vi "SIAM_test_Standalone.vi"() -> ()   [LabVIEW 2011]
uses:
  SIAM_command.ctl
  Library/ScanControl/ScanControl_Action.ctl
  Library/ScanControl/ScanControl_Channel.ctl
  SIAM-send.ctl
  <vilib>/Utility/miscctls.llb/LVRangeTypeDef.ctl
panel:
  in  "Registerkarte":enum32{"Config", "Scan", "Work", "Debug"}(tab)
  out "Instrument check":bool
  in  "expected instrument name":string="Earn_Out"
  in  "TMSI-device-scales":T2(array[cluster])=[{"channel"=enum."GalvoX", "m/bit"=8e-07, "min m"=-0.01, "max m"=0.01, "max a [m/s]"=1.0}, {"channel"=enum."GalvoY", "m/bit"=8e-07, "min m"=-0.01, "max m"=0.01, "max a [m/s]"=1.0}, {"channel"=enum."Galvo3", "m/bit"=2e-09, "min m"=-0.01, "max m"=0.02, "max a [m/s]"=1.0}]
  out "Connected":bool
  in  "remote port or service name":u16=3
  in  "address":string="10.153.70.119"
  out "connect error":errorcluster
  in  "Cycletime [s]":dbl=1e-05
  in  "Update length":bool
  out "Elements":i32
  in  "Unroll-loops":bool
  in  "ClearScan":bool
  in  "channel":T1=enum."GalvoX"
  in  "ConvertScan":bool
  in  "Convert String":bool
  in  "Colibri-Scan-String":string="0,0,10,0.00119;0,0,3,-7.2266666667E-5;0,0,4,-8.8133333333E-5;0,0,11,0;0,0,12,0;0,0,7,3;0,4,9,127;0,2,3,0.05875;0,2,4,0;0,2,11,100000;0.00255,2,11,0;0.00256,1,12,1;0.00256,0,7,1;0.00256,2,3,-1.4928955695E-16;0.00256,2,4,0.0073046875;0.00264,0,7,3;0.00264,2,3,-0.05875;0.00264,2,4,0;0.00264,2,11,-100000;0.00519,2,11,0;0.0052,1,12,1;0.0052,0,7,1;0.0052,2,3,1.4928955695E-16;0.0052,2,4,0.0073046875;0.00528,0,7,3;0.00528,5,9,0;0.67056,2,3,0.05875;0.67056,2,4,0;0.67056,2,11,100000;0.67311,2,11,0;0.67312,1,12,1;0.67312,0,7,1;0.67312,2,3,-1.4928955695E-16;0.67312,2,4,0.0073046875;0.6732,0,7,3;0.6732,2,3,-0.05875;0.6732,2,4,0;0.6732,2,11,-100000;0.67575,2,11,0;0.67576,2,3,0;0.67576,2,4,0;0.67576,0,7,0;"
  in  "ScanSteuerung":T4(array[cluster])
  in  "Frequency [Hz]":dbl=500.0
  in  "duration [s]":dbl=1.0
  in  "Amplitude (count pk-pk)":dbl=6553.6 format="%#_5g"
  in  "Create":bool
  in  "Offset [count]":dbl=1.0
  in  "Run":bool
  in  "SendScript":bool
  in  "Load":bool
  in  "Save":bool
  in  "ClearScript":bool
  in  "Value":i32
  in  "Motor":T5(ring)
  in  "Position":i32(slide)
  in  "Clear":bool
  in  "Special":bool
  in  "return":string
  in  "special send options":T6
  in  "Script":T8(array[cluster])=[{"Delay 10µs"=0, "command"=100663297, "P0"=1024, "P1"=-2147483648, "P2"=0, "P3"=0, "P4"=0, "P5-ticket"=0}, {"Delay 10µs"=0, "command"=100663297, "P0"=16384, "P1"=2147483647, "P2"=0, "P3"=0, "P4"=0, "P5-ticket"=0}, {"Delay 10µs"=0, "command"=100663297, "P0"=512, "P1"=2147483647, "P2"=0, "P3"=0, "P4"=0, "P5-ticket"=0}, {"Delay 10µs"=0, "command"=100663297, "P0"=8192, "P1"=0, "P2"=0, "P3"=0, "P4"=0, "P5-ticket"=0}, {"Delay 10µs"=119, "command"=4060086273, "P0"=2, "P1"=99, "P2"=0, "P3"=0, "P4"=0, "P5-ticket"=0}, {"Delay 10µs"=0, "command"=218103809, "P0"=255, "P1"=7, "P2"=0, "P3"=0, "P4"=0, "P5-ticket"=0}, {"Delay 10µs"=281, "command"=100663297, "P0"=512, "P1"=0, "P2"=0, "P3"=0, "P4"=0, "P5-ticket"=0}, {"Delay 10µs"=0, "command"=100663297, "P0"=8192, "P1"=-2147483648, "P2"=0, "P3"=0, "P4"=0, "P5-ticket"=0}, {"Delay 10µs"=8, "command"=100663297, "P0"=512, "P1"=-2147483648, "P2"=0, "P3"=0, "P4"=0, "P5-ticket"=0}, {"Delay 10µs"=0, "command"=100663297, "P0"=8192, "P1"=0, "P2"=0, "P3"=0, "P4"=0, "P5-ticket"=0}, {"Delay 10µs"=111, "command"=218103809, "P0"=255, "P1"=5, "P2"=0, "P3"=0, "P4"=0, "P5-ticket"=0}, {"Delay 10µs"=8, "command"=218103809, "P0"=255, "P1"=7, "P2"=0, "P3"=0, "P4"=0, "P5-ticket"=0}, {"Delay 10µs"=281, "command"=100663297, "P0"=512, "P1"=0, "P2"=0, "P3"=0, "P4"=0, "P5-ticket"=0}, {"Delay 10µs"=0, "command"=100663297, "P0"=8192, "P1"=-2147483648, "P2"=0, "P3"=0, "P4"=0, "P5-ticket"=0}, {"Delay 10µs"=8, "command"=100663297, "P0"=512, "P1"=2147483647, "P2"=0, "P3"=0, "P4"=0, "P5-ticket"=0}, {"Delay 10µs"=0, "command"=100663297, "P0"=8192, "P1"=0, "P2"=0, "P3"=0, "P4"=0, "P5-ticket"=0}, {"Delay 10µs"=111, "command"=218103809, "P0"=255, "P1"=5, "P2"=0, "P3"=0, "P4"=0, "P5-ticket"=0}, {"Delay 10µs"=8, "command"=4043375201, "P0"=-12, "P1"=2, "P2"=1, "P3"=0, "P4"=0, "P5-ticket"=0}, {"Delay 10µs"=0, "command"=218103809, "P0"=255, "P1"=7, "P2"=0, "P3"=0, "P4"=0, "P5-ticket"=0}, {"Delay 10µs"=281, "command"=100663297, "P0"=512, "P1"=0, "P2"=0, "P3"=0, "P4"=0, "P5-ticket"=0}, {"Delay 10µs"=0, "command"=100663297, "P0"=8192, "P1"=-2147483648, "P2"=0, "P3"=0, "P4"=0, "P5-ticket"=0}, {"Delay 10µs"=8, "command"=100663297, "P0"=512, "P1"=-2147483648, "P2"=0, "P3"=0, "P4"=0, "P5-ticket"=0}, {"Delay 10µs"=0, "command"=100663297, "P0"=8192, "P1"=0, "P2"=0, "P3"=0, "P4"=0, "P5-ticket"=0}, {"Delay 10µs"=111, "command"=218103809, "P0"=255, "P1"=5, "P2"=0, "P3"=0, "P4"=0, "P5-ticket"=0}, {"Delay 10µs"=8, "command"=218103809, "P0"=255, "P1"=7, "P2"=0, "P3"=0, "P4"=0, "P5-ticket"=0}, {"Delay 10µs"=281, "command"=100663297, "P0"=512, "P1"=0, "P2"=0, "P3"=0, "P4"=0, "P5-ticket"=0}, {"Delay 10µs"=0, "command"=100663297, "P0"=8192, "P1"=0, "P2"=0, "P3"=0, "P4"=0, "P5-ticket"=0}, {"Delay 10µs"=0, "command"=4060086273, "P0"=2, "P1"=4, "P2"=0, "P3"=0, "P4"=0, "P5-ticket"=0}, {"Delay 10µs"=1, "command"=100663297, "P0"=1024, "P1"=-2147483648, "P2"=0, "P3"=0, "P4"=0, "P5-ticket"=0}, {"Delay 10µs"=0, "command"=100663297, "P0"=16384, "P1"=2147483647, "P2"=0, "P3"=0, "P4"=0, "P5-ticket"=0}, {"Delay 10µs"=0, "command"=100663297, "P0"=512, "P1"=2147483647, "P2"=0, "P3"=0, "P4"=0, "P5-ticket"=0}, {"Delay 10µs"=0, "command"=100663297, "P0"=8192, "P1"=0, "P2"=0, "P3"=0, "P4"=0, "P5-ticket"=0}, {"Delay 10µs"=118, "command"=218103809, "P0"=255, "P1"=4, "P2"=0, "P3"=0, "P4"=0, "P5-ticket"=0}, {"Delay 10µs"=1, "command"=4060086273, "P0"=3, "P1"=99, "P2"=0, "P3"=0, "P4"=0, "P5-ticket"=0}, {"Delay 10µs"=0, "command"=218103809, "P0"=255, "P1"=7, "P2"=0, "P3"=0, "P4"=0, "P5-ticket"=0}, {"Delay 10µs"=281, "command"=100663297, "P0"=512, "P1"=0, "P2"=0, "P3"=0, "P4"=0, "P5-ticket"=0}, {"Delay 10µs"=0, "command"=100663297, "P0"=8192, "P1"=-2147483648, "P2"=0, "P3"=0, "P4"=0, "P5-ticket"=0}, {"Delay 10µs"=8, "command"=100663297, "P0"=512, "P1"=-2147483648, "P2"=0, "P3"=0, "P4"=0, "P5-ticket"=0}, {"Delay 10µs"=0, "command"=100663297, "P0"=8192, "P1"=0, "P2"=0, "P3"=0, "P4"=0, "P5-ticket"=0}, {"Delay 10µs"=111, "command"=218103809, "P0"=255, "P1"=5, "P2"=0, "P3"=0, "P4"=0, "P5-ticket"=0}, {"Delay 10µs"=8, "command"=218103809, "P0"=255, "P1"=7, "P2"=0, "P3"=0, "P4"=0, "P5-ticket"=0}, {"Delay 10µs"=281, "command"=100663297, "P0"=512, "P1"=0, "P2"=0, "P3"=0, "P4"=0, "P5-ticket"=0}, {"Delay 10µs"=0, "command"=100663297, "P0"=8192, "P1"=-2147483648, "P2"=0, "P3"=0, "P4"=0, "P5-ticket"=0}, {"Delay 10µs"=8, "command"=100663297, "P0"=512, "P1"=2147483647, "P2"=0, "P3"=0, "P4"=0, "P5-ticket"=0}, {"Delay 10µs"=0, "command"=100663297, "P0"=8192, "P1"=0, "P2"=0, "P3"=0, "P4"=0, "P5-ticket"=0}, {"Delay 10µs"=111, "command"=218103809, "P0"=255, "P1"=5, "P2"=0, "P3"=0, "P4"=0, "P5-ticket"=0}, {"Delay 10µs"=8, "command"=4043375201, "P0"=-12, "P1"=3, "P2"=1, "P3"=0, "P4"=0, "P5-ticket"=0}, {"Delay 10µs"=0, "command"=218103809, "P0"=255, "P1"=7, "P2"=0, "P3"=0, "P4"=0, "P5-ticket"=0}, {"Delay 10µs"=281, "command"=100663297, "P0"=512, "P1"=0, "P2"=0, "P3"=0, "P4"=0, "P5-ticket"=0}, {"Delay 10µs"=0, "command"=100663297, "P0"=8192, "P1"=-2147483648, "P2"=0, "P3"=0, "P4"=0, "P5-ticket"=0}, {"Delay 10µs"=8, "command"=100663297, "P0"=512, "P1"=-2147483648, "P2"=0, "P3"=0, "P4"=0, "P5-ticket"=0}, {"Delay 10µs"=0, "command"=100663297, "P0"=8192, "P1"=0, "P2"=0, "P3"=0, "P4"=0, "P5-ticket"=0}, {"Delay 10µs"=111, "command"=218103809, "P0"=255, "P1"=5, "P2"=0, "P3"=0, "P4"=0, "P5-ticket"=0}, {"Delay 10µs"=8, "command"=218103809, "P0"=255, "P1"=7, "P2"=0, "P3"=0, "P4"=0, "P5-ticket"=0}, {"Delay 10µs"=281, "command"=100663297, "P0"=512, "P1"=0, "P2"=0, "P3"=0, "P4"=0, "P5-ticket"=0}, {"Delay 10µs"=0, "command"=100663297, "P0"=8192, "P1"=0, "P2"=0, "P3"=0, "P4"=0, "P5-ticket"=0}, {"Delay 10µs"=0, "command"=4043375201, "P0"=-28, "P1"=2, "P2"=1, "P3"=0, "P4"=0, "P5-ticket"=0}, {"Delay 10µs"=119, "command"=218103809, "P0"=255, "P1"=0, "P2"=0, "P3"=0, "P4"=0, "P5-ticket"=0}, {"Delay 10µs"=0, "command"=4027518991, "P0"=0, "P1"=0, "P2"=0, "P3"=0, "P4"=0, "P5-ticket"=0}] {"command" format="%x" items=["read_x-Motor_status_ticket"=17305600, "init_x-Motor"=17760263, "read_x-Motor_absolute_ticket"=16781312, "move_x-Motor_absolute"=16777217, "move_x-Motor_relative"=16842753, "read_y-Motor_status_ticket"=18354176, "init_y-Motor"=18808839, "read_y-Motor_absolute_ticket"=17829888, "move_y-Motor_absolute"=17825793, "move_y-Motor_relative"=17891329, "read_z-Motor_status_ticket"=19402752, "init_z-Motor"=19857415, "stop_z-Motor"=19857423, "start_z-Motor"=19857422, "read_z-Motor_absolute_ticket"=18878464, "move_z-Motor_absolute"=18874369, "move_z-Motor_relative"=18939905, "end_no_ticket"=4027514895, "end_ticket"=4027518991, "IO-read_bank0"=3489665024, "IO-write_bank0"=3489660929, "IO-read_bank1"=3506442240, "IO-write_bank1"=3506438145, "Analog-write_DA0-0"=2684354561, "Analog-write_DA0-1"=2685403137, "Analog-write_DA0-2"=2686451713, "Analog-write_DA0-3"=2687500289, "Analog-write_DA0-4"=2688548865, "Analog-write_DA0-5"=2689597441, "Analog-write_DA0-6"=2690646017, "Analog-write_DA0-7"=2691694593, "Analog-write_DA1-0"=2701131777, "Analog-write_DA1-1"=2702180353, "Analog-write_DA1-2"=2703228929, "Analog-write_DA1-3"=2704277505, "Analog-write_DA1-4"=2705326081, "Analog-write_DA1-5"=2706374657, "Analog-write_DA1-6"=2707423233, "Analog-write_DA1-7"=2708471809, "Analog-read_AD0-0"=2818576384, "Analog-read-store_AD0-0"=2818572290, "IO-delay_bank0"=3489923073, "IO-delay_bank0_fromVar"=3489923075, "read_cam_clock"=3289124864, "store_cam_clock"=3289120770, "read_cam_phase"=3289190400, "set_cam_deadtime"=3288989697, "set_cam_10uscycles"=3289055233, "set_cam_10uscycles_fromVariable"=3289055235, "calc_cam"=3289317386, "store_cam_Var"=3289251842, "math_addToVariable"=4060086278, "readVar"=4060090368, "writeVar"=4060086273, "copyVar"=4060086276, "decrement_branchRel_if_equal"=4043374945, "decrement_branchRel_if_greaterequal"=4043375201, "decrement_branchRel_if_greaterequal_withTicket"=4043379297, "decrement_branchRel_if_smaller"=4043375457, "increment_branchRel_if_smaller"=4043375473, "set_x-Galvo"=1612710129, "set_y-Galvo"=1613758705, "set_z-Fokus"=1614807281, "set_x-Galvo_position-only"=1612709953, "set_y-Galvo_position-only"=1613758529, "set_z-Fokus_position-only"=1614807105, "set_x-Galvo_position-only_ticket"=1612714049, "set_y-Galvo_position-only_ticket"=1613762625, "set_z-Fokus_position-only_ticket"=1614811201, "set_x-Galvo_speed-only"=1612709921, "set_y-Galvo_speed-only"=1613758497, "set_z-Fokus_speed-only"=1614807073, "read_x-Galvo_ticket"=1612714048, "read_y-Galvo_ticket"=1613762624, "read_z-Focus_ticket"=1614811200, "x-Galvo_pos_fromVar"=1612709955, "y-Galvo_pos_fromVar"=1613758531, "z-Focus_pos_fromVar"=1614807107]; "P5-ticket" format="%.0x"; "Delay 10µs" format="%.0x"; "P0" format="%.0x"; "P1" format="%.0x"}
  out "String":string
  in  "Ignore Connect Error (test conversion etc)":bool
  out "Return":i32[](array[numeric]) format="%.0x"
  out "send error":errorcluster
  out "recieve error":errorcluster
  in  "MotorScale":cluster{"Scale.Range":T9, "Value":i32}[](array[cluster])=[{"Scale.Range"={"Minimum"=-32000.0, "Maximum"=32000.0, "Increment"=50000.0, "Minor Increment"=5000.0, "Start"=0.0}, "Value"=0}, {"Scale.Range"={"Minimum"=-32000.0, "Maximum"=32000.0, "Increment"=50000.0, "Minor Increment"=5000.0, "Start"=0.0}, "Value"=3557}, {"Scale.Range"={"Minimum"=7000.0, "Maximum"=28000.0, "Increment"=10000.0, "Minor Increment"=2000.0, "Start"=10000.0}, "Value"=9970}, {"Scale.Range"={"Minimum"=-32000.0, "Maximum"=32000.0, "Increment"=50000.0, "Minor Increment"=5000.0, "Start"=0.0}, "Value"=0}, {"Scale.Range"={"Minimum"=-2667000.0, "Maximum"=-2660000.0, "Increment"=7000.0, "Minor Increment"=500.0, "Start"=-2667000.0}, "Value"=-2660919}]
  in  "End":bool
  # "enter before execution"
  # "better this constants, for each device?\nGalvo +-30°opt,f=50mm: 7.9897E-7 m/count"
  # "TMSI-Direkt:"
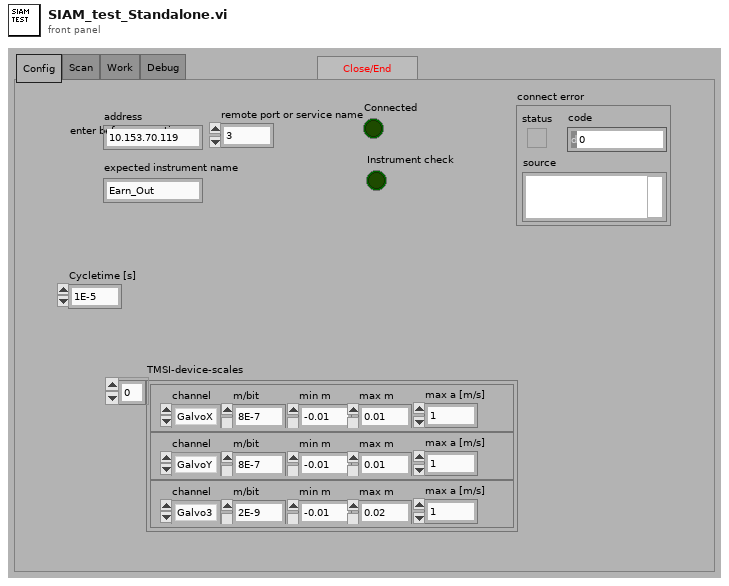
[diagram p1: front panel]
types:
  T1 = typedef "ScanControl_Channel.ctl" = enum16{"Com", "AnalogConfig", "AnalogValue", "GalvoX", "GalvoY", "Galvo3", "Galvo4", "Digital", "Free", "Loop", "SMoveTime", "Image1X", "Image1Y", "Image2X", "Image2Y"}
  T2 = cluster{"channel":T1, "m/bit":dbl, "min m":dbl, "max m":dbl, "max a [m/s]":dbl}[]
  T3 = typedef "ScanControl_Action.ctl" = enum16{"Abs", "Rel", "Inc", "IncInc", "LoopStart", "LoopEnd", "WaitTriggerRising"}
  T4 = cluster{"Time [s]":dbl, "action":T3, "channel":T1, "value (m/s)":dbl}[]
  T5 = enum16{"Ch0", "Ch1", "x-Galvo", "y-Galvo", "z-Focus"}
  T6 = typedef "SIAM-send.ctl" = enum16{"validID", "storeID", "enable", "rundirect", "sendlist", "run", "stop", "readRegister", "sendValue", "storeStatus"}
  T7 = typedef "SIAM_command.ctl" = u32
  T8 = cluster{"Delay 10µs":u32, "command":T7, "P0":i32, "P1":i32, "P2":i32, "P3":i32, "P4":i32, "P5-ticket":i32}[]
  T9 = typedef "LVRangeTypeDef.ctl" = cluster{"Minimum":dbl, "Maximum":dbl, "Increment":dbl, "Minor Increment":dbl, "Start":dbl}
  T10 = enum16{"Standard", "Buffered", "CRLF", "Immediate"}
  T11 = cluster{"rel 10µs":u32, "Device":T7, "data0":i32, "data1":i32, "data2":i32, "data3":i32, "data4":i32, "data5":i32}
  T12 = enum16{"triangle", "fixed xy-circle", "fixed xy-square"}
  T13 = cluster{"Time [s]":dbl, "action":T3, "channel":T1, "value (/s)":dbl}[]
  T14 = cluster{"rel 10µs":u32, "Device":T7, "data0":i32, "data1":i32, "data2":i32, "data3":i32, "data4":i32, "data5":i32}[]
  T15 = typedef "ScanControl.ctl" = cluster{"Time [s]":dbl, "action":T3, "channel":T1, "value (/s)":dbl}[]
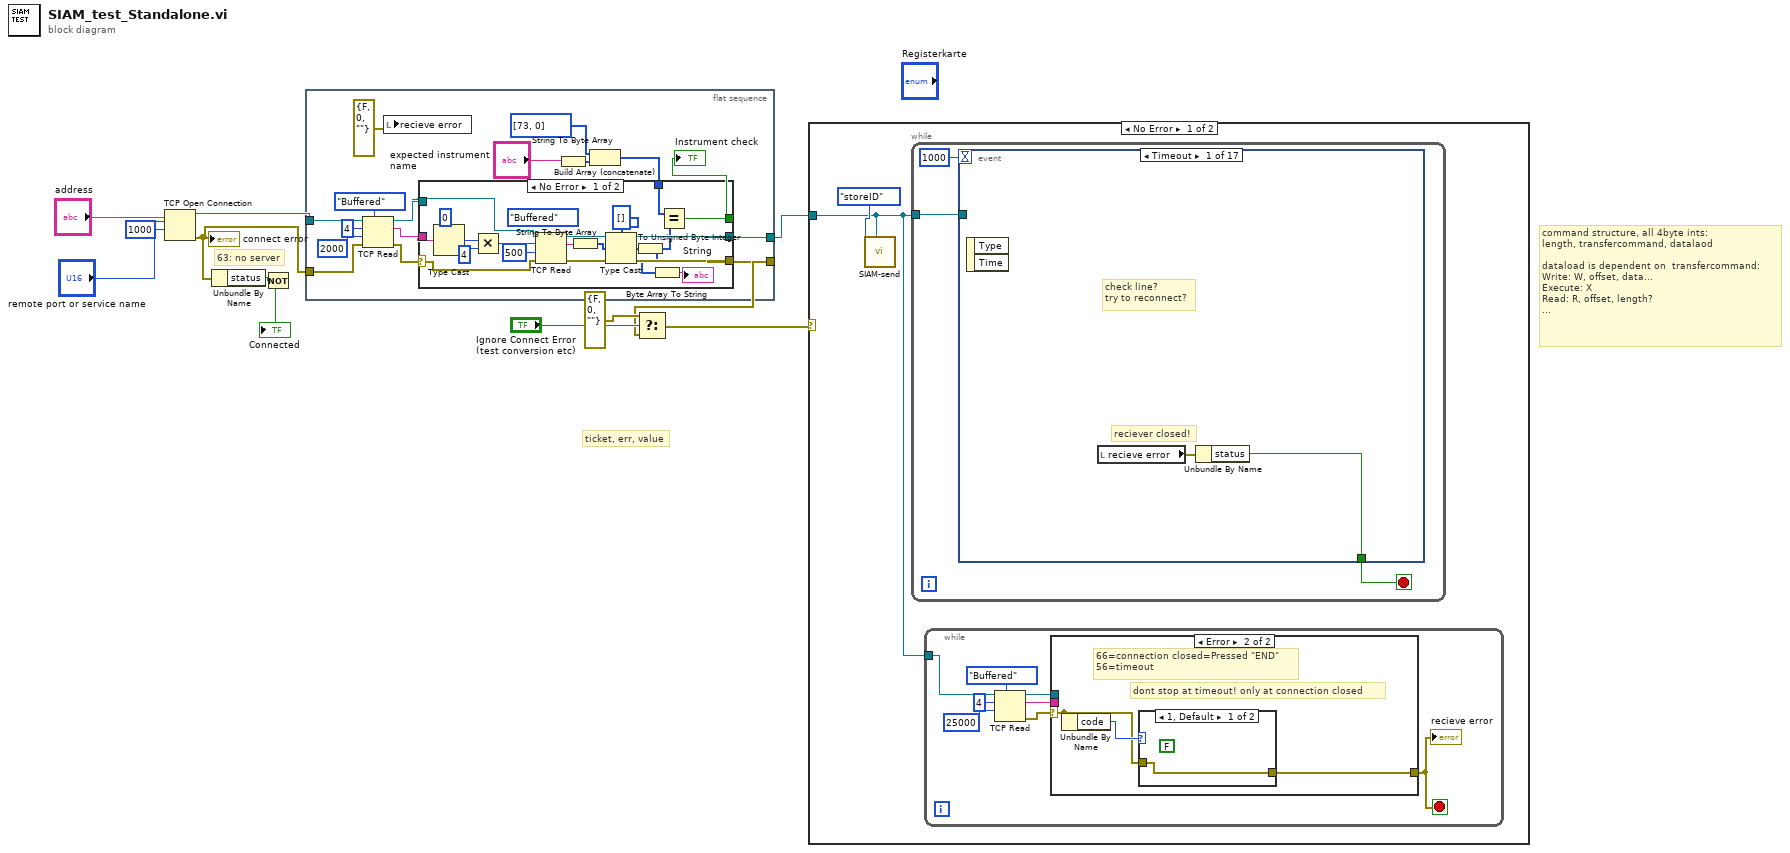
[diagram p0: block diagram]
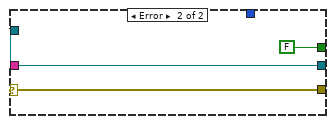
[diagram p2: hidden frame]
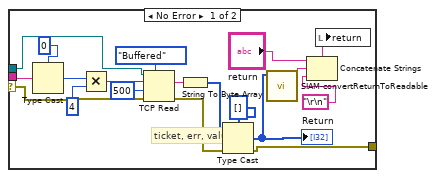
[diagram p3: hidden frame]
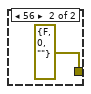
[diagram p4: hidden frame]
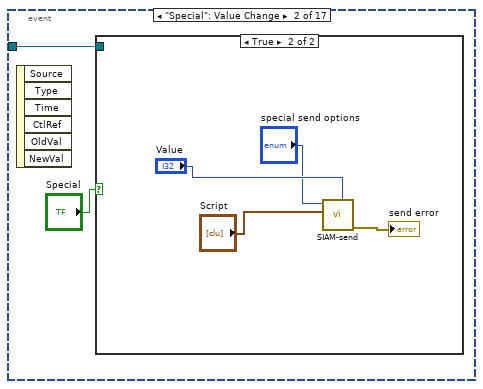
[diagram p5: hidden frame]
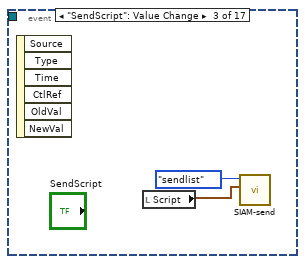
[diagram p7: hidden frame]
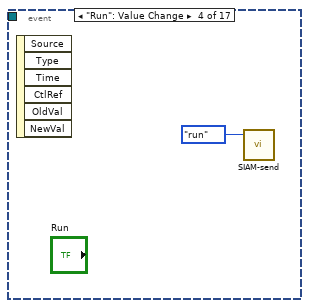
[diagram p8: hidden frame]
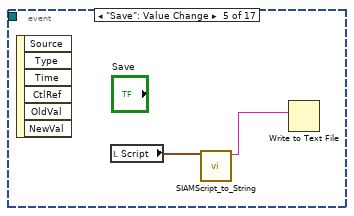
[diagram p9: hidden frame]
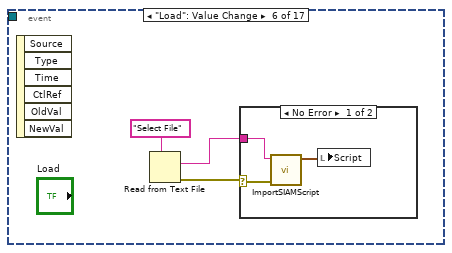
[diagram p10: hidden frame]
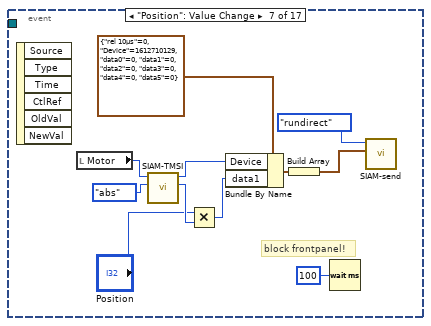
[diagram p12: hidden frame]
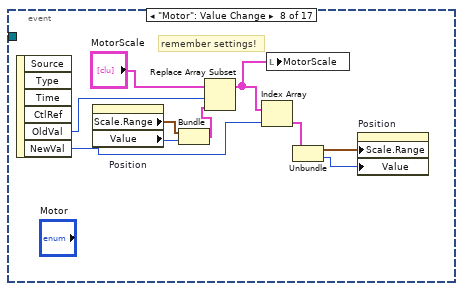
[diagram p13: hidden frame]
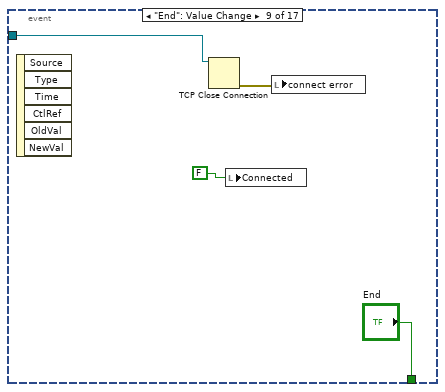
[diagram p14: hidden frame]
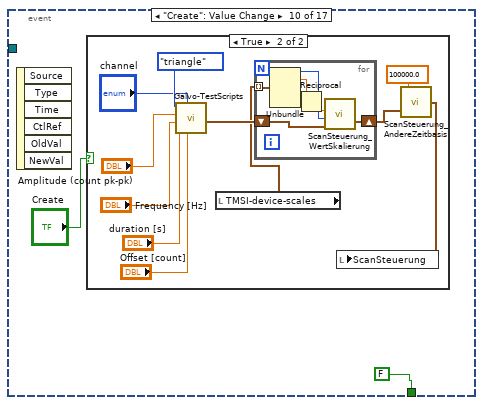
[diagram p15: hidden frame]
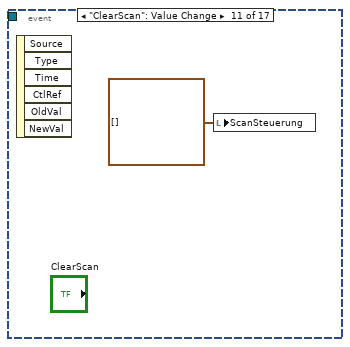
[diagram p17: hidden frame]
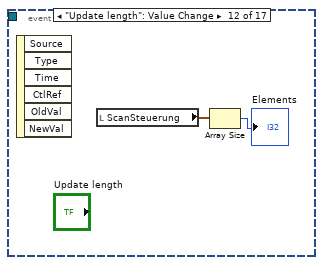
[diagram p18: hidden frame]
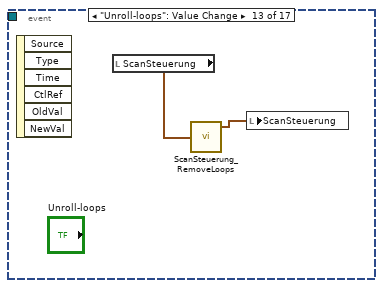
[diagram p19: hidden frame]
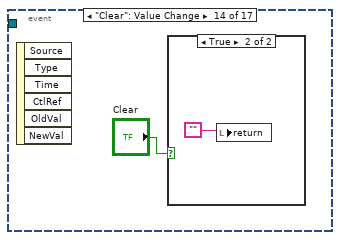
[diagram p20: hidden frame]
diagram:
  # "ticket, err, value"
  # "63: no server"
  # "command structure, all 4byte ints:\nlength, transfercommand, datalaod\n\ndataload is dependent on  transfercommand:\nWrite: W, offset, data...\nExecute: X\nRead: R, offset, length?\n..."
  n1 = TCP Open Connection(address="address", remote port or service name="remote port or service name", timeout ms (60000)=1000) -> (connection ID=w2:refnum<k5>, error out=w4:errorcluster)  [unwired: 1 in, 1 out]
  "connect error" <- w4
  n2 = Unbundle By Name(w4) -> ("status"=w10:bool)
  n3 = Not(x=w10) -> (.not. x?=→"Connected":bool)
  n4 = flat-sequence {
    tunnel: w2 -> [w19]
    tunnel: w4 -> [w22]
    tunnel: [w21] -> w3
    tunnel: [w20] -> w1
    frame #0 {
      n5 = TCP Read(connection ID=w19, bytes to read=4, error in (no error)=w22, 7:T10."Buffered" ("mode (standard)"), 9:2000 ("timeout ms (25000)")) -> (connection ID out=w24:refnum<k5>, data out=w23:string, error out=w25:errorcluster)
      n6 = local write "recieve error"(errorcluster {"status"=FALSE, "code"=0, "source"=""} ("recieve error")) -> ()
      n7 = String To Byte Array(string="expected instrument name") -> (unsigned byte array=w18:u8[])
      n8 = Build Array (concatenate)(u8[] [73, 0] ("element"), w18) -> (w15:u8[])
      n9 = case shown="No Error" w25 {
        selector: w25 -> [w40 w49]
        tunnel: w24 -> [w41 w48]
        tunnel: w23 -> [w39 _]
        tunnel: [w38 w49] -> w21
        tunnel: [w37 w48] -> w20
        tunnel: w15 -> [w32 _]
        tunnel: [w31 FALSE] -> w14
        frame No Error {
          (unwired) T10."Buffered" ("mode (standard)")
          n10 = Type Cast(type=u32 0, x=w39) -> (*(type *) &x=w44:u32)
          n11 = Multiply(x=w44, y=u32 4) -> (x*y=w46:u32)
          n12 = TCP Read(connection ID=w41, bytes to read=w46, error in (no error)=w40, 9:500 ("timeout ms (25000)")) -> (connection ID out=w37:refnum<k5>, data out=w34:string, error out=w38:errorcluster)  [unwired: 1 in]
          n13 = String To Byte Array(string=w34) -> (unsigned byte array=w35:u8[])
          n14 = Type Cast(type=i32[] [], x=w35) -> (*(type *) &x=w33:i32[])
          n15 = To Unsigned Byte Integer(number=w33) -> (unsigned 8bit integer=w30:u8[])
          n16 = Byte Array To String(unsigned byte array=w30) -> (string=→"String":string)
          n17 = Equal?(x=w32, y=w30) -> (x = y?=w31:bool)
        }
        frame Error {
        }
      }
      "Instrument check" <- w14
    }
  }
  n18 = Select(t=errorcluster {"status"=FALSE, "code"=0, "source"=""}, s="Ignore Connect Error (test conversion etc)", f=w3) -> (s? t:f=w7:errorcluster)
  n19 = case shown="No Error" w7 {
    tunnel: w1 -> [w50 _]
    frame No Error {
      n20 = call "SIAM-send.vi"("connection ID"=w50, "command"=SIAM-send."storeID") -> ()  [unwired: 8 in, 2 out]
      n21 = while {
        tunnel: w50 -> [w84]
        stop <- w85 stop-if-true
        n22 = event shown="[0] Timeout" {
          selector: _ -> [_ _ _ _ _ _ _ _ _ _ _ _ _ _ _ _ _]
          dyn-events: _ -> [_ _ _ _ _ _ _ _ _ _ _ _ _ _ _ _ _]
          timeout: 1000 -> [_ _ _ _ _ _ _ _ _ _ _ _ _ _ _ _ _]
          tunnel: [w86 _ _ _ _ _ _ _ "End" FALSE _ _ _ _ _ _ _] -> w85
          tunnel: w84 -> [_ w88 _ _ _ _ _ _ w128 _ _ _ _ _ _ _ _]
          event Timeout {
            # "reciever closed!"
            # "check line?\ntry to reconnect?"
            n23 = event-data() -> ()  [unwired: 3 out]
            n24 = local read "recieve error"() -> (w87:errorcluster)
            n25 = Unbundle By Name(w87) -> ("status"=w86:bool)
          }
          event "Special": Value Change {
            n26 = event-data() -> ()  [unwired: 7 out]
            n27 = case shown="True" "Special" {
              tunnel: w88 -> [_ _]
              frame False {
              }
              frame True {
                n28 = call "SIAM-send.vi"("Value"="Value", "Script"="Script", "command"="special send options") -> ("error out"=→"send error":errorcluster)  [unwired: 7 in, 1 out]
              }
            }
          }
          event "SendScript": Value Change {
            n29 = event-data() -> ()  [unwired: 7 out]
            n30 = local read "Script"() -> (w95:T8)
            n31 = call "SIAM-send.vi"("Script"=w95, "command"=SIAM-send."sendlist") -> ()  [unwired: 8 in, 2 out]
          }
          event "Run": Value Change {
            n32 = event-data() -> ()  [unwired: 7 out]
            n33 = call "SIAM-send.vi"("command"=SIAM-send."run") -> ()  [unwired: 9 in, 2 out]
          }
          event "Save": Value Change {
            n34 = event-data() -> ()  [unwired: 7 out]
            n35 = local read "Script"() -> (w98:T8)
            n36 = call "SIAMScript_to_String.vi"("Script"=w98) -> ("String"=w97:string)  [unwired: 9 in, 1 out]
            n37 = Write to Text File(text=w97) -> ()  [unwired: 3 in, 3 out]
          }
          event "Load": Value Change {
            n38 = event-data() -> ()  [unwired: 7 out]
            n39 = Read from Text File(prompt (Open existing file)="Select File") -> (text=w100:string, error out=w99:errorcluster)  [unwired: 3 in, 2 out]
            n40 = case shown="No Error" w99 {
              selector: w99 -> [w102 _]
              tunnel: w100 -> [w103 _]
              frame No Error {
                n41 = call "ImportSIAMScript.vi"("error in (no error)"=w102, "String"=w103) -> ("Script"=w104:T8)  [unwired: 8 in, 1 out]
                n42 = local write "Script"(w104) -> ()
              }
              frame Error {
              }
            }
          }
          event "Position": Value Change {
            # "block frontpanel!"
            n43 = event-data() -> ()  [unwired: 7 out]
            n44 = local read "Motor"() -> (w105:T5)
            n45 = call "SIAM-TMSI.vi"("Type"=enum8{"acc", "vel", "abs", "offset"}."abs", "Motor"=w105) -> ("Resolution-Factor"=w111:i32, "command"=w107:T7)  [unwired: 6 in, 2 out]
            n46 = Multiply(x="Position", y=w111) -> (x*y=w109:i32)
            n47 = Bundle By Name(cluster=T11 {"rel 10µs"=0, "Device"=1612710129, "data0"=0, "data1"=0, "data2"=0, "data3"=0, "data4"=0, "data5"=0} ("output cluster"), "Device"=w107, "data1"=w109) -> (w115:T11)
            n48 = Build Array(w115) -> (w114:T14)
            n49 = Wait (ms)(milliseconds to wait=u32 100) -> ()  [unwired: 1 out]
            n50 = call "SIAM-send.vi"("Script"=w114, "command"=SIAM-send."rundirect") -> ()  [unwired: 8 in, 2 out]
          }
          event "Motor": Value Change {
            # "remember settings!"
            n51 = event-data() -> ("OldVal"=w125:T5, "NewVal"=w124:T5)  [unwired: 5 out]
            n52 = property on="Position" class="Slide (strict)"() -> ("Scale.Range"=w121:T9, "Value"=w122:i32)  [unwired: 2 in, 2 out]
            n53 = Bundle("Scale.Range"=w121, "Value"=w122) -> (w120:cluster{"Scale.Range":T9, "Value":i32})  [unwired: 1 in]
            n54 = Replace Array Subset(array="MotorScale", new element=w120, index=w125) -> (w118:cluster{"Scale.Range":T9, "Value":i32}[])
            n55 = Index Array(array=w118, index=w124) -> (element=w123:cluster{"Scale.Range":T9, "Value":i32})
            n56 = local write "MotorScale"(w118) -> ()
            n57 = Unbundle(w123) -> ("Scale.Range"=w117:T9, "Value"=w116:i32)
            n58 = property on="Position" class="Slide (strict)"("Scale.Range"=w117, "Value"=w116) -> ()  [unwired: 2 in, 2 out]
          }
          event "End": Value Change {
            n59 = event-data() -> ()  [unwired: 7 out]
            n60 = TCP Close Connection(connection ID=w128) -> (error out=w127:errorcluster)  [unwired: 1 in, 2 out]
            n61 = local write "Connected"(FALSE ("Connected")) -> ()
            n62 = local write "connect error"(w127) -> ()
          }
          event "Create": Value Change {
            n63 = event-data() -> ()  [unwired: 7 out]
            n64 = case shown="True" "Create" {
              frame False {
              }
              frame True {
                n65 = call "Galvo-TestScripts.vi"("Type"=T12."triangle", "channel"="channel", "Amplitude"="Amplitude (count pk-pk)", "Frequency[Hz]"="Frequency [Hz]", "Offset"="Offset [count]", "Duration [s]"="duration [s]") -> ("ScanSteuerung"=w134:T15)  [unwired: 1 in, 1 out]
                n66 = local read "TMSI-device-scales"() -> (w132:T2)
                n67 = for {
                  shift-right: [w147] -> w133
                  shift-left: w134 -> [w148]
                  tunnel: w132 -> [w146] mode=indexing
                  n68 = Unbundle(w146) -> ("channel"=w145:T1, "m/bit"=w144:dbl)  [unwired: 3 out]
                  n69 = Reciprocal(x=w144) -> (1/x=w143:dbl)
                  n70 = call "ScanSteuerung_WertSkalierung.vi"("ScanSteuerung"=w148, "Channel"=w145, "/Skalierung (m/bit)"=w143) -> ("ScanSteuerungOut"=w147:T15)  [unwired: 1 in]
                }
                n71 = call "ScanSteuerung_AndereZeitbasis.vi"("ScanSteuerung"=w133, "Neues Zeitraster"=100000.0) -> ("ScanSteuerungOut"=w135:T15)
                n72 = local write "ScanSteuerung"(w135) -> ()
              }
            }
          }
          event "ClearScan": Value Change {
            n73 = event-data() -> ()  [unwired: 7 out]
            n74 = local write "ScanSteuerung"(T13 [] ("ScanSteuerung")) -> ()
          }
          event "Update length": Value Change {
            n75 = event-data() -> ()  [unwired: 7 out]
            n76 = local read "ScanSteuerung"() -> (w151:T4)
            n77 = Array Size(array=w151) -> (size(s)=→"Elements":i32)
          }
          event "Unroll-loops": Value Change {
            n78 = event-data() -> ()  [unwired: 7 out]
            n79 = local read "ScanSteuerung"() -> (w153:T4)
            n80 = call "ScanSteuerung_RemoveLoops.vi"("ScanSteuerung"=w153) -> ("ScanSteuerungOut"=w152:T15)  [unwired: 2 out]
            n81 = local write "ScanSteuerung"(w152) -> ()
          }
          event "Clear": Value Change {
            n82 = event-data() -> ()  [unwired: 7 out]
            n83 = case shown="True" "Clear" {
              frame False {
              }
              frame True {
                n84 = local write "return"("") -> ()
              }
            }
          }
          event "ClearScript": Value Change {
            n85 = event-data() -> ()  [unwired: 7 out]
            n86 = local write "Script"(T8 [] ("Script")) -> ()
          }
          event "ConvertScan": Value Change {
            n87 = event-data() -> ()  [unwired: 7 out]
            n88 = call "ScanSteuerung_AndereZeitbasis.vi"("ScanSteuerung"="ScanSteuerung", "Neues Zeitraster"="Cycletime [s]") -> ("ScanSteuerungOut"=w160:T15)
            n89 = for {
              shift-right: [w166] -> w158
              shift-left: w160 -> [w167]
              tunnel: "TMSI-device-scales" -> [w165] mode=indexing
              n90 = Unbundle(w165) -> ("channel"=w164:T1, "m/bit"=w163:dbl)  [unwired: 3 out]
              n91 = call "ScanSteuerung_WertSkalierung.vi"("ScanSteuerung"=w167, "Channel"=w164, "/Skalierung (m/bit)"=w163) -> ("ScanSteuerungOut"=w166:T15)  [unwired: 1 in]
            }
            n92 = call "ScanControl_to_SIAM.vi"("ScanSteuerung"=w158) -> ("Script"=w161:T8)  [unwired: 1 in, 9 out]
            n93 = local write "Script"(w161) -> ()
          }
          event "Convert String": Value Change {
            n94 = event-data() -> ()  [unwired: 7 out]
            n95 = call "String2ScanSteuerung.vi"("String"="Colibri-Scan-String") -> ("ScanSteuerung"=w168:T15)
            n96 = local write "ScanSteuerung"(w168) -> ()
          }
        }
      }
      n97 = while {
        tunnel: w50 -> [w59]
        stop <- w52 stop-if-true
        n98 = TCP Read(connection ID=w59, bytes to read=4, 7:T10."Buffered" ("mode (standard)"), 9:25000 ("timeout ms (25000)")) -> (connection ID out=w55:refnum<k5>, data out=w56:string, error out=w53:errorcluster)  [unwired: 1 in]
        n99 = case shown="Error" w53 {
          selector: w53 -> [w73 w78]
          tunnel: w56 -> [w77 _]
          tunnel: w55 -> [w74 _]
          tunnel: [w63 w79] -> w52
          frame No Error {
            # "ticket, err, value"
            n100 = Type Cast(type=u32 0, x=w77) -> (*(type *) &x=w66:u32)
            n101 = Multiply(x=w66, y=u32 4) -> (x*y=w64:u32)
            n102 = TCP Read(connection ID=w74, bytes to read=w64, error in (no error)=w73, 7:T10."Buffered" ("mode (standard)"), 9:500 ("timeout ms (25000)")) -> (data out=w71:string, error out=w63:errorcluster)  [unwired: 1 out]
            n103 = String To Byte Array(string=w71) -> (unsigned byte array=w67:u8[])
            n104 = Type Cast(type=i32[] [], x=w67) -> (*(type *) &x=w60:i32[])
            "Return" <- w60
            n105 = call "SIAM-convertReturnToReadable.vi"("Return"=w60) -> ("Readable"=w68:string)  [unwired: 1 in, 9 out]
            n106 = Concatenate Strings("return", w68, "\r\n") -> (w70:string)
            n107 = local write "return"(w70) -> ()
          }
          frame Error {
            # "dont stop at timeout! only at connection closed"
            # "66=connection closed=Pressed \"END\"\n56=timeout"
            n108 = Unbundle By Name(w78) -> ("code"=w80:i32)
            n109 = case shown="1, Default" w80 {
              tunnel: [w81 errorcluster {"status"=FALSE, "code"=0, "source"=""} ("error out")] -> w79
              tunnel: w78 -> [w81 _]
              frame 1, Default {
                (unwired) FALSE ("Connected")
              }
              frame 56 {
              }
            }
          }
        }
        "recieve error" <- w52
      }
    }
    frame Error {
    }
  }
